vi "initializeStyle.vi"(8 "error in (no error)":errorcluster, 10 "Style":refnum<class "Style.lvclass">, 11 "xwpfRun.Title in":refnum<class "xwpfRun.Title.lvclass">) -> (0 "error out":errorcluster, 3 "xwpfRun.Title out":refnum<class "xwpfRun.Title.lvclass">)   [LabVIEW 2017, in "Word_Specific.lvlib" / "xwpfRun.Title.lvclass"]
uses:
  xwpfRun.Title.lvclass
  Styles/Style/Style.lvclass
  Styles/Title/Title.lvclass
  C:/Users/Neo/Desktop/Dev_Tools_BR/LabVIEW_NPOI/src/Styles/Style/Style.lvclass
  xwpfRun/xwpfRun.lvclass
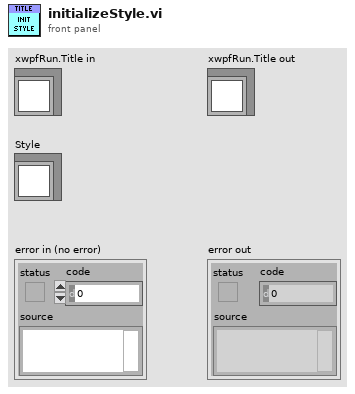
[diagram p1: front panel]
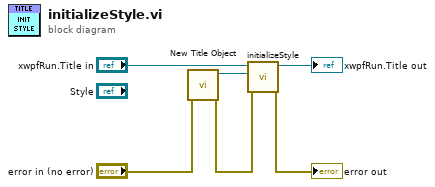
[diagram p0: block diagram]
diagram:
  n1 = call "New Title Object.vi"("error in (no error)"="error in (no error)") -> ("error out"=w2:errorcluster, "Title out"=w3:refnum<class "Title.lvclass">)  [unwired: 9 in]
  n2 = call-parent "initializeStyle.vi"("error in (no error)"=w2, "Style"=w3, "xwpfRun in"="xwpfRun.Title in") -> ("error out"=→"error out":errorcluster, "xwpfRun out"=→"xwpfRun.Title out":refnum<class "xwpfRun.Title.lvclass">)  [unwired: 7 in]
